vi "IMAQdx Reset Ethernet Camera Address.vi"(7 "Timeout (1000 ms)":u32=1000, 8 "error in":errorcluster, 10 "Camera Address (0.0.0.0)":T1={"Address"="0.0.0.0", "Subnet"="0.0.0.0", "Gateway"="0.0.0.0"}, 11 "Session In":T2) -> (0 "error out":errorcluster)   [LabVIEW 2020, in "NI_Vision_Acquisition_Software.lvlib"]
doc: "Reset Ethernet camera address. Use this function to reset Ethernet cameras on the network with a local subnet. This function will be blocked and will return when the reset is complete or after the specified timeout."
uses:
  NI_Vision_Acquisition_Software.lvlib
  IMAQdx.ctl
  niimaqdx.dll
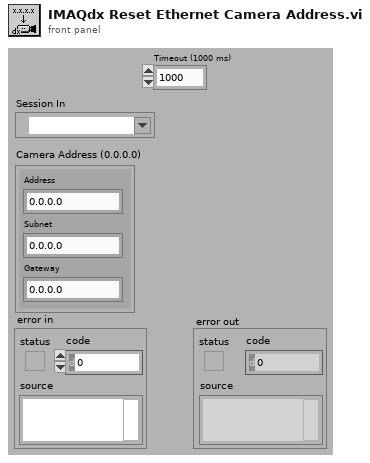
[diagram p1: front panel]
types:
  T1 = cluster{"Address":string, "Subnet":string, "Gateway":string}
  T2 = typedef "IMAQdx.ctl" = refnum<k21>
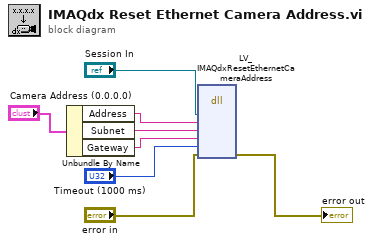
[diagram p0: block diagram]
diagram:
  n1 = Unbundle By Name("Camera Address (0.0.0.0)") -> ("Address"=w3:string, "Subnet"=w2:string, "Gateway"=w1:string)
  n2 = dll-call lib="niimaqdx.dll" fn="LV_IMAQdxResetEthernetCameraAddress"("name"="Session In", "address"=w3, "subnet"=w2, "gateway"=w1, "timeout"="Timeout (1000 ms)", "error in"="error in") -> ("error in"=→"error out":errorcluster)  [unwired: 9 in, 2 out]
